vi "Send Message.vi"(7 "Data DVR":refnum<data-value>, 8 "error in (no error)":errorcluster, 11 "Notify with Message in":refnum<class "Notify With Data.lvclass">) -> (0 "error out":errorcluster, 3 "Notify with Message out":refnum<class "Notify With Data.lvclass">)   [LabVIEW 2023, in "Notify With Data.lvclass"]
uses:
  Notify With Data.lvclass
  Data/Data.lvclass
  Controls/User Event Operations.ctl
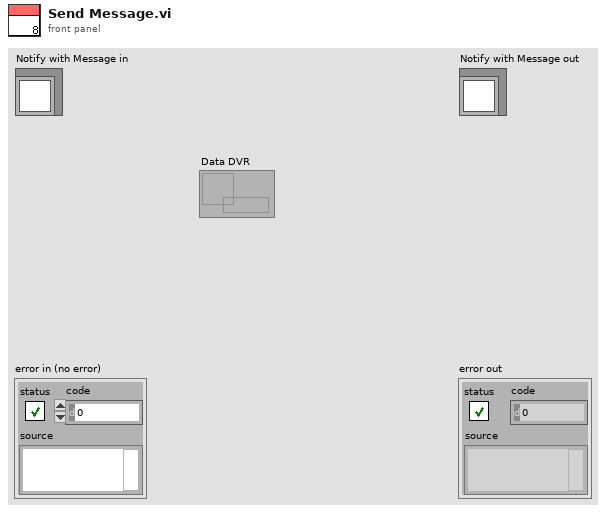
[diagram p1: front panel]
types:
  T1 = typedef "User Event Operations.ctl" = enum16{"Obtain", "Generate", "Destroy"}
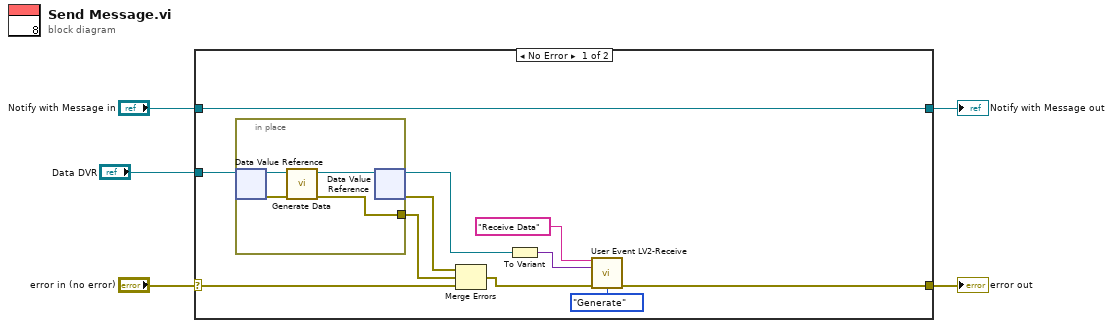
[diagram p0: block diagram]
diagram:
  n1 = case shown="No Error" "error in (no error)" {
    selector: "error in (no error)" -> [w16 w22]
    tunnel: [w8 w22] -> w4
    tunnel: [w7 w21] -> w2
    tunnel: "Notify with Message in" -> [w7 w21]
    tunnel: "Data DVR" -> [w15 _]
    frame No Error {
      n2 = in-place {
        in-place-border: [w17] -> w13
        n3 = in-place-dvr #1(w15) -> (w19:refnum<class "Data.lvclass">, w20:errorcluster)
        n4 = call-dynamic "Generate Data.vi"("Error In"=w20, "Data in"=w19) -> ("Error Out"=w17:errorcluster, "Data out"=w18:refnum<class "Data.lvclass">)  [unwired: 8 in]
        n5 = in-place-dvr #1(w18) -> (w6:refnum<data-value>, w14:errorcluster)
      }
      n6 = Merge Errors(w14, w13, w16) -> (w9:errorcluster)
      n7 = To Variant(anything=w6) -> (Variant=w10:variant)
      n8 = call "User Event LV2-Receive.vi"("Event Name"="Receive Data", "Data"=w10, "Error In"=w9, "Operation"=User_Event_Operations."Generate") -> ("Error Out"=w8:errorcluster)  [unwired: 10 in, 1 out]
    }
    frame Error {
    }
  }
  "error out" <- w4
  "Notify with Message out" <- w2
